vi "Process.vi"(8 "error in":errorcluster, 11 "Plugin in":refnum<class "Waterfall.lvclass">) -> (0 "error out":errorcluster, 3 "Plugin out":refnum<class "Waterfall.lvclass">)   [LabVIEW 2024, in "Waterfall.lvlib" / "Waterfall.lvclass"]
uses:
  Waterfall.lvclass
  Waterfall.lvclass/Waterfall.ctl
  <vilib>/FlexLogger/SDK/PluginSDK.lvlibp/PEFClasses/SDK/Plugin/Plugin.lvclass
  C:/Program Files/National Instruments/LabVIEW 2024/vi.lib/FlexLogger/SDK/PluginSDK.lvlibp/PEFClasses/SDK/Plugin/Plugin.lvclass
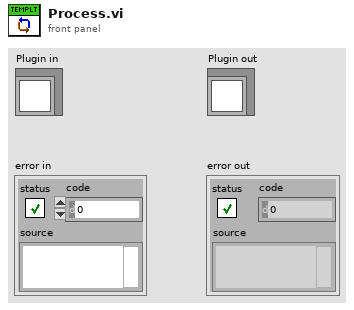
[diagram p1: front panel]
types:
  T1 = typedef "Waterfall.lvlib/Waterfall.lvclass/Waterfall Data.ctl" = cluster{"First Time":bool, "Show Waterfall Button Clicked":bool, "Data to Process":dbl, "Slice":dbl, "window":T2, "averaging parameters":cluster{"averaging mode":enum16{"No averaging", "Vector averaging", "RMS averaging", "Peak hold"}, "weighting mode":enum16{"Linear", "Exponential"}, "number of averages":u32}, "Waterfall VI Ref":refnum<vi>, "Signal":waveform(dbl)}
  T2 = typedef "NI_AALPro.lvlib/windowTd.ctl" = u32
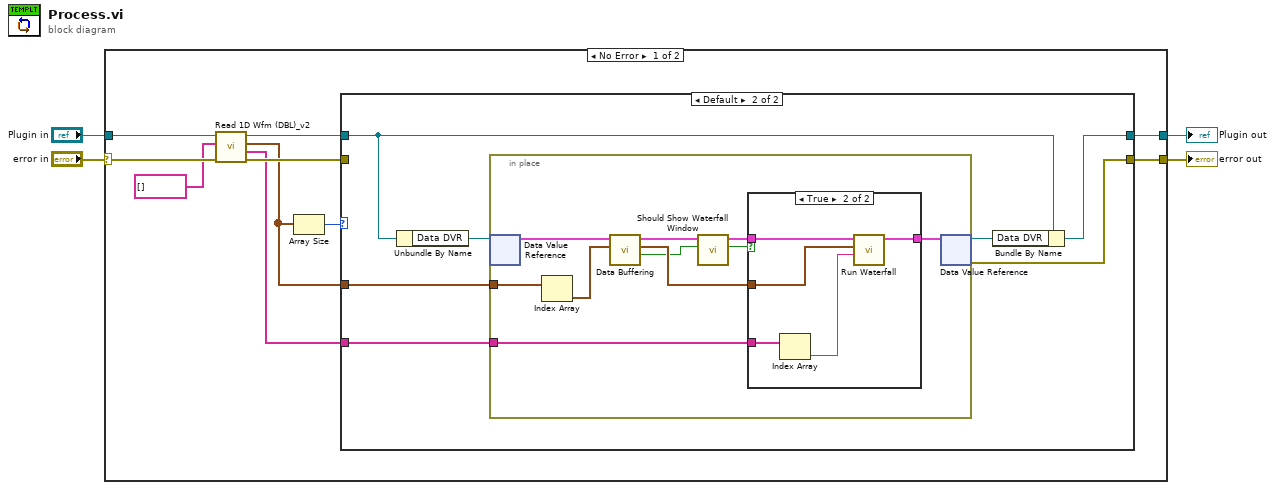
[diagram p0: block diagram]
diagram:
  n1 = case shown="No Error" "error in" {
    selector: "error in" -> [w13 w40]
    tunnel: [w5 w41] -> w1
    tunnel: "Plugin in" -> [w14 w41]
    tunnel: [w12 w40] -> w2
    frame No Error {
      n2 = call <vilib>:"Read 1D Wfm (DBL)_v2.vi"("error in (no error)"=w13, "Unique Identifers (empty = all)"=string[] [] ("Unique Channel Identifers (empty = all)"), "Plugin in"=w14) -> ("error out"=w10:errorcluster, "Stream Names"=w8:string[], "Data"=w7:waveform(dbl)[], "Plugin out"=w6:refnum<class "Waterfall.lvclass">)  [unwired: 5 in]
      n3 = Array Size(array=w7) -> (size(s)=w11:i32)
      n4 = case shown="Default" w11 {
        tunnel: w7 -> [_ w23]
        tunnel: [w16 w17] -> w12
        tunnel: w10 -> [w16 _]
        tunnel: w8 -> [_ w22]
        tunnel: w6 -> [w15 w19]
        tunnel: [w15 w18] -> w5
        frame 0 {
          # "No channels sending data to the plugin"
        }
        frame Default {
          n5 = Unbundle By Name(w19) -> ("Data DVR"=w21:refnum<data-value>)
          n6 = in-place {
            in-place-border: w23 -> [w32]
            in-place-border: w22 -> [w33]
            n7 = in-place-dvr #1(w21) -> (w26:T1)  [unwired: 1 out]
            n8 = Index Array(array=w32) -> (element=w31:waveform(dbl))  [unwired: 1 in]
            n9 = call "Data Buffering.vi"("Signal"=w31, "Data in"=w26) -> ("Data Ready"=w27:bool, "Data to Process"=w30:waveform(dbl), "Data out"=w28:T1)  [unwired: 7 in]
            n10 = call "Should Show Waterfall Window.vi"("Data Valid"=w27, "Data in"=w28) -> ("Show Window"=w25:bool, "Data out"=w24:T1)  [unwired: 8 in]
            n11 = case shown="True" w25 {
              tunnel: w24 -> [w34 w38]
              tunnel: [w34 w36] -> w29
              tunnel: w33 -> [_ w39]
              tunnel: w30 -> [_ w35]
              frame False {
              }
              frame True {
                n12 = Index Array(array=w39) -> (element=w37:string)  [unwired: 1 in]
                n13 = call "Run Waterfall.vi"("Channel Name"=w37, "Signal"=w35, "Data"=w38) -> ("Data dup"=w36:T1)  [unwired: 8 in]
              }
            }
            n14 = in-place-dvr #1(w29) -> (w20:refnum<data-value>, w17:errorcluster)
          }
          n15 = Bundle By Name(cluster=w19, "Data DVR"=w20) -> (w18:refnum<class "Waterfall.lvclass">)
        }
      }
    }
    frame Error {
    }
  }
  "error out" <- w2
  "Plugin out" <- w1
